vi "Incremental Moving Average.vi"(8 "error in (no error)":errorcluster, 10 "Reset (F)":bool, 11 "Value":dbl) -> (0 "error out":errorcluster, 1 "Iterations":dbl, 2 "Total":dbl, 3 "Average":dbl)   [LabVIEW 2011]
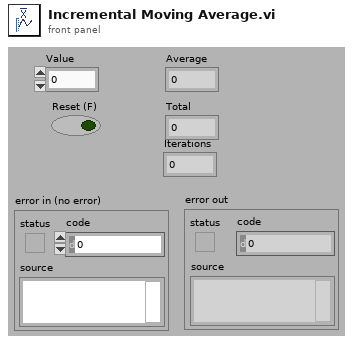
[diagram p1: front panel]
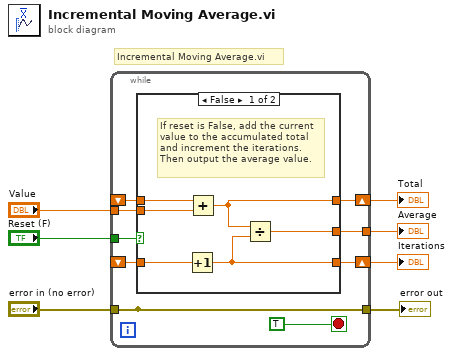
[diagram p0: block diagram]
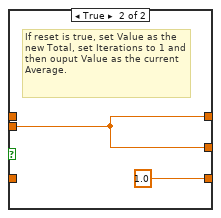
[diagram p2: hidden frame]
diagram:
  # "Incremental Moving Average.vi"
  n1 = while {
    shift-right: [w12] -> w5
    shift-left: _ -> [w15]
    tunnel: "Value" -> [w14]
    shift-right: [w11] -> w4
    shift-left: _ -> [w13]
    tunnel: "Reset (F)" -> [w10]
    tunnel: [w9] -> w3
    tunnel: [w8] -> _
    tunnel: "error in (no error)" -> [w8]
    tunnel: [w8] -> w1
    stop <- TRUE stop-if-true
    n2 = case shown="False" w10 {
      tunnel: w15 -> [w22 _]
      tunnel: w14 -> [w21 w24]
      tunnel: w13 -> [w20 _]
      tunnel: [w19 w24] -> w12
      tunnel: [w18 1.0] -> w11
      tunnel: [w17 w24] -> w9
      frame False {
        # "If reset is False, add the current value to the accumulated total and increment the iterations.  Then output the average value."
        n3 = Increment(x=w20) -> (x+1=w18:dbl)
        n4 = Add(x=w22, y=w21) -> (x+y=w19:dbl)
        n5 = Divide(x=w19, y=w18) -> (x/y=w17:dbl)
      }
      frame True {
        # "If reset is true, set Value as the new Total, set Iterations to 1 and then ouput Value as the current Average."
      }
    }
  }
  "Total" <- w5
  "Iterations" <- w4
  "Average" <- w3
  "error out" <- w1
